vi "Get_Parameter Json.vi"(8 "error in (no error)":errorcluster caption="entrée d'erreur (pas d'erreur)", 11 "Class Instrument Relay_Board en entrée":refnum<class "Class Instrument UART.lvclass">) -> (0 "error out":errorcluster caption="sortie d'erreur", 2 "Parameter Json":string, 3 "Class Instrument Relay_Board en sortie":refnum<class "Class Instrument UART.lvclass">)   [LabVIEW 2020, in "Library Instrument & Equipement.lvlib" / "Library Instruments.lvlib" / "Class Instrument UART.lvclass"]
uses:
  Class Instrument UART.lvclass
  Class Instrument UART.lvclass/Class Instrument UART.ctl
  JSON API/Variant JSON/Variant to JSON.vi
  JSON API/JSON Value/Get Item by name array.vi
  Instrument (Default)/Class Instrument (Default).lvclass
  JSON API/JSON Value/JSON Value.lvclass
  JSON API/Get Polymorphic/JSON GetSet.lvlib
  JSON API/Variant JSON/Variant JSON.lvlib
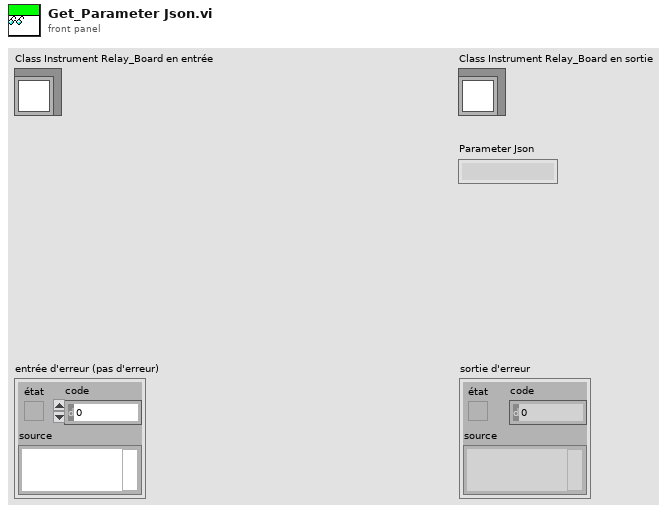
[diagram p1: front panel]
types:
  T1 = typedef "Parametre UART.ctl" = cluster{"Address Device":refnum<visa-resource-name>, "Baud Rate":u32, "Data Bit":u16, "stop bits (10: 1 bit)":u16, "parity (0:none)":enum16{"None", "Odd", "Even", "Mark", "Space"}, "flow control (0:none)":u16, "termination char ":u8, "Enable Termination":bool, "Nb Octet to Read":u16, "Class UART":refnum<class "Class UART (Default).lvclass">}
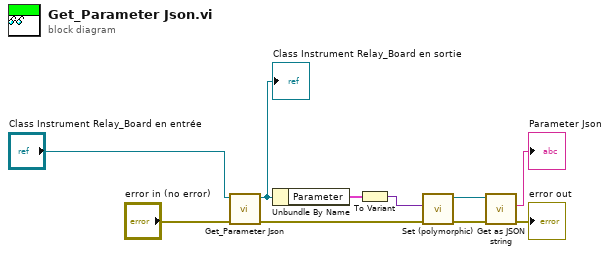
[diagram p0: block diagram]
diagram:
  n1 = call-parent "Get_Parameter Json.vi"("error in (no error)"="error in (no error)", "Class Instrument (Default) en entrée"="Class Instrument Relay_Board en entrée") -> ("error out"=w4:errorcluster, "Class Instrument (Default) en sortie"=w2:refnum<class "Class Instrument UART.lvclass">)  [unwired: 7 in, 1 out]
  "Class Instrument Relay_Board en sortie" <- w2
  n2 = Unbundle By Name(w2) -> ("Parameter"=w1:T1)
  n3 = To Variant(anything=w1) -> (Variant=w8:variant)
  n4 = call-poly "Set (polymorphic).vi"("error in (no error)"=w4, "Variant"=w8) -> ("error out"=w6:errorcluster, "JSON Value out"=w7:refnum<class "JSON Value.lvclass">)  [unwired: 8 in]
  n5 = call "Get as JSON string.vi"("error in (no error)"=w6, "JSON Value in"=w7) -> ("error out"=→"error out":errorcluster, "<JSON>"=→"Parameter Json":string)  [unwired: 8 in]
